vi "3global.vi"() -> ()   [LabVIEW 2026]
panel:
  in  "Stop global":bool
  in  "Data":dbl[][](array[numeric])
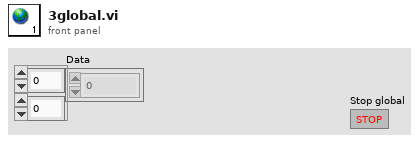
[diagram p1: front panel]
diagram:
